vi "日志存储 (子VI).vi"(11 "data in":T1) -> ()   [LabVIEW 2016, in "数据传输系统-02.lvlib"]
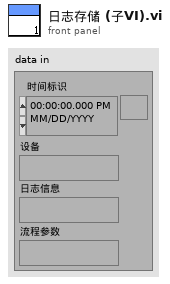
[diagram p1: front panel]
types:
  T1 = cluster{"时间标识":timestamp, "设备":string, "日志信息":string, "流程参数":string}
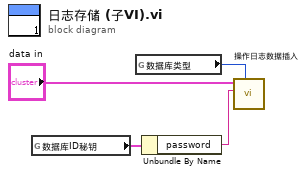
[diagram p0: block diagram]
diagram:
  n1 = global read "外部交互全局.vi" "数据库ID秘钥"() -> (w2:cluster{"userID":string, "password":string})
  n2 = global read "断电保存全局.vi" "数据库类型"() -> (w3:enum16{"Access", "SQLite"})
  n3 = Unbundle By Name(w2) -> ("password"=w1:string)
  n4 = call "操作日志数据插入.vi"("data"="data in", "Password"=w1, "数据库类型"=w3) -> ()  [unwired: 7 in, 1 out]
